vi "hw3-2 topVI.vi"() -> ()   [LabVIEW 2014]
panel:
  out "input":dbl[](array[numeric])
  out "XY Graph":cluster{i32[], dbl[]}(graph)
  out "temp":dbl[](array[numeric])
  out "sorted":dbl[](array[numeric])
  out "Max":u32
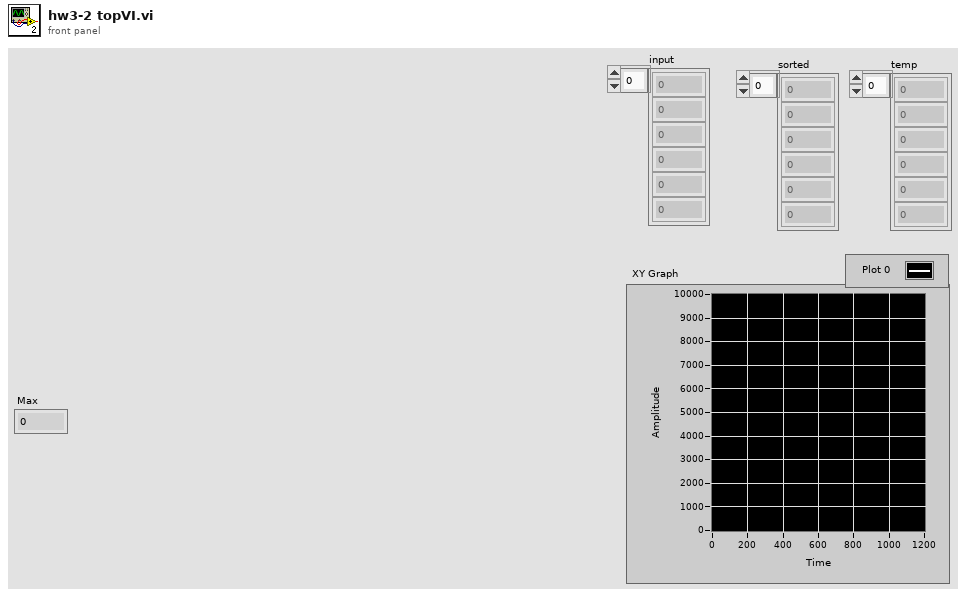
[diagram p1: front panel]
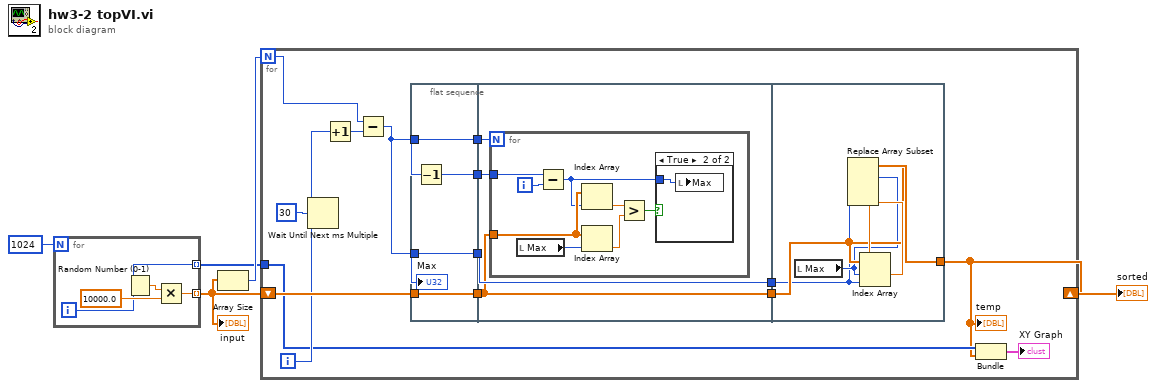
[diagram p0: block diagram]
diagram:
  n1 = for {
    N: 1024 -> [_]
    tunnel: [w7] -> w2 mode=indexing
    tunnel: [w6] -> w1 mode=indexing
    i -> [w6]
    n2 = Random Number (0-1)() -> (number: 0 to 1=w9:dbl)
    n3 = Multiply(x=w9, y=10000.0) -> (x*y=w7:dbl)
  }
  "input" <- w2
  n4 = Array Size(array=w2) -> (size(s)=w5:i32)
  n5 = for {
    N: w5 -> [w14]
    shift-right: [w10] -> w4
    shift-left: w2 -> [w24]
    tunnel: w1 -> [w11]
    i -> [w16]
    n6 = Wait Until Next ms Multiple(millisecond multiple=u32 30) -> ()  [unwired: 1 out]
    n7 = Increment(x=w16) -> (x+1=w15:i32)
    n8 = Subtract(x=w14, y=w15) -> (x-y=w17:i32)
    n9 = flat-sequence {
      tunnel: w24 -> [w28]
      tunnel: [w28] -> w23
      tunnel: w17 -> [w25]
      tunnel: [w27] -> w20
      tunnel: w17 -> [w27]
      tunnel: [w26] -> w19
      tunnel: [w25] -> w13
      tunnel: w23 -> [w30]
      tunnel: [w30] -> w22
      tunnel: [w32] -> w21
      tunnel: w20 -> [w32]
      tunnel: w19 -> [w31]
      tunnel: w13 -> [w29]
      tunnel: w22 -> [w44]
      tunnel: w21 -> [w42]
      tunnel: [w45] -> w10
      frame #0 {
        n10 = Decrement(x=w25) -> (x-1=w26:i32)
        "Max" <- w27
      }
      frame #1 {
        n11 = for {
          N: w29 -> [_]
          tunnel: w30 -> [w39]
          tunnel: w31 -> [w35]
          i -> [w34]
          n12 = local read "Max"() -> (w40:u32)
          n13 = Subtract(x=w35, y=w34) -> (x-y=w33:i32)
          n14 = Index Array(array=w39, index=w33) -> (element=w37:dbl)
          n15 = Index Array(array=w39, index=w40) -> (element=w36:dbl)
          n16 = Greater?(x=w37, y=w36) -> (0:w38:bool)
          n17 = case shown="True" w38 {
            tunnel: w33 -> [_ w41]
            frame False {
            }
            frame True {
              n18 = local write "Max"(w41) -> ()
            }
          }
        }
      }
      frame #2 {
        n19 = local read "Max"() -> (w43:u32)
        n20 = Index Array(array=w44, index #1=w43, index #2=w42) -> (element #1=w46:dbl, element #2=w47:dbl)
        n21 = Replace Array Subset(array=w44, new element #1=w47, index #1=w43, new element #2=w46, index #2=w42) -> (w45:dbl[])
      }
    }
    n22 = Bundle(w11, w10) -> (→"XY Graph":cluster{i32[], dbl[]})  [unwired: 1 in]
    "temp" <- w10
  }
  "sorted" <- w4
